vi "Main program.vi"() -> ()   [LabVIEW 2020]
panel:
  in  "stop":bool
  out "Final Amount":dbl format="$%#_g"
  in  "Calculate":bool
  in  "Compounded":string(combo)
  in  "Year":dbl min=0.0 max=100.0
  in  "Interest rate":dbl format="%.2f%"
  in  "Investment":dbl format="$%#_g"
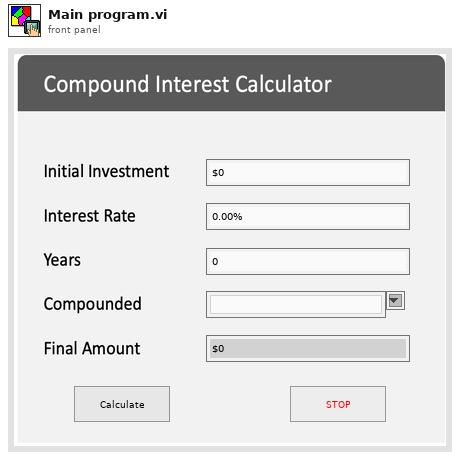
[diagram p1: front panel]
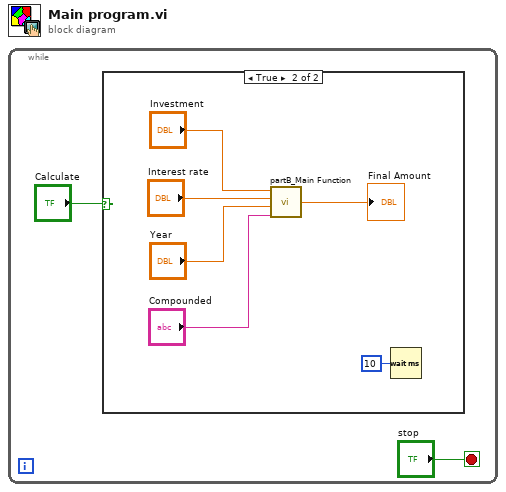
[diagram p0: block diagram]
diagram:
  n1 = while {
    stop <- "stop" stop-if-true
    n2 = case shown="True" "Calculate" {
      frame False {
      }
      frame True {
        n3 = call "partB_Main Function.vi"("Compounded"="Compounded", "Year"="Year", "Interest rate"="Interest rate", "Investment"="Investment") -> ("Final Amount"=→"Final Amount":dbl)
        n4 = Wait (ms)(milliseconds to wait=u32 10) -> ()  [unwired: 1 out]
      }
    }
  }
